vi "timemer.vi"() -> ()   [LabVIEW 2014]
panel:
  out "문자열":string
  in  "확인 버튼 2":bool
  in  "초기화":bool
  in  "확인 버튼":bool
  out "초":i32[](array[numeric])
  out "분":i32[](array[numeric])
  out "시":i32[](array[numeric])
  out "시간":string
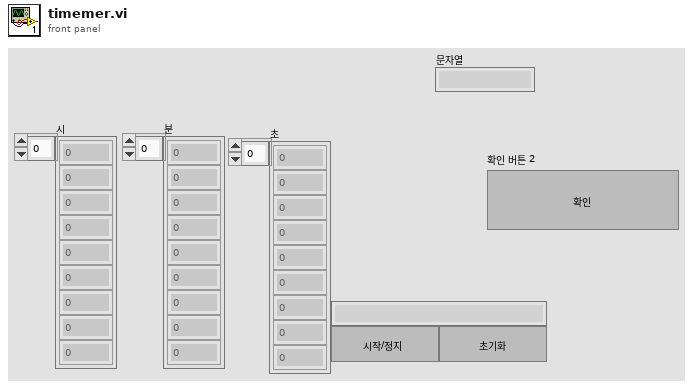
[diagram p1: front panel]
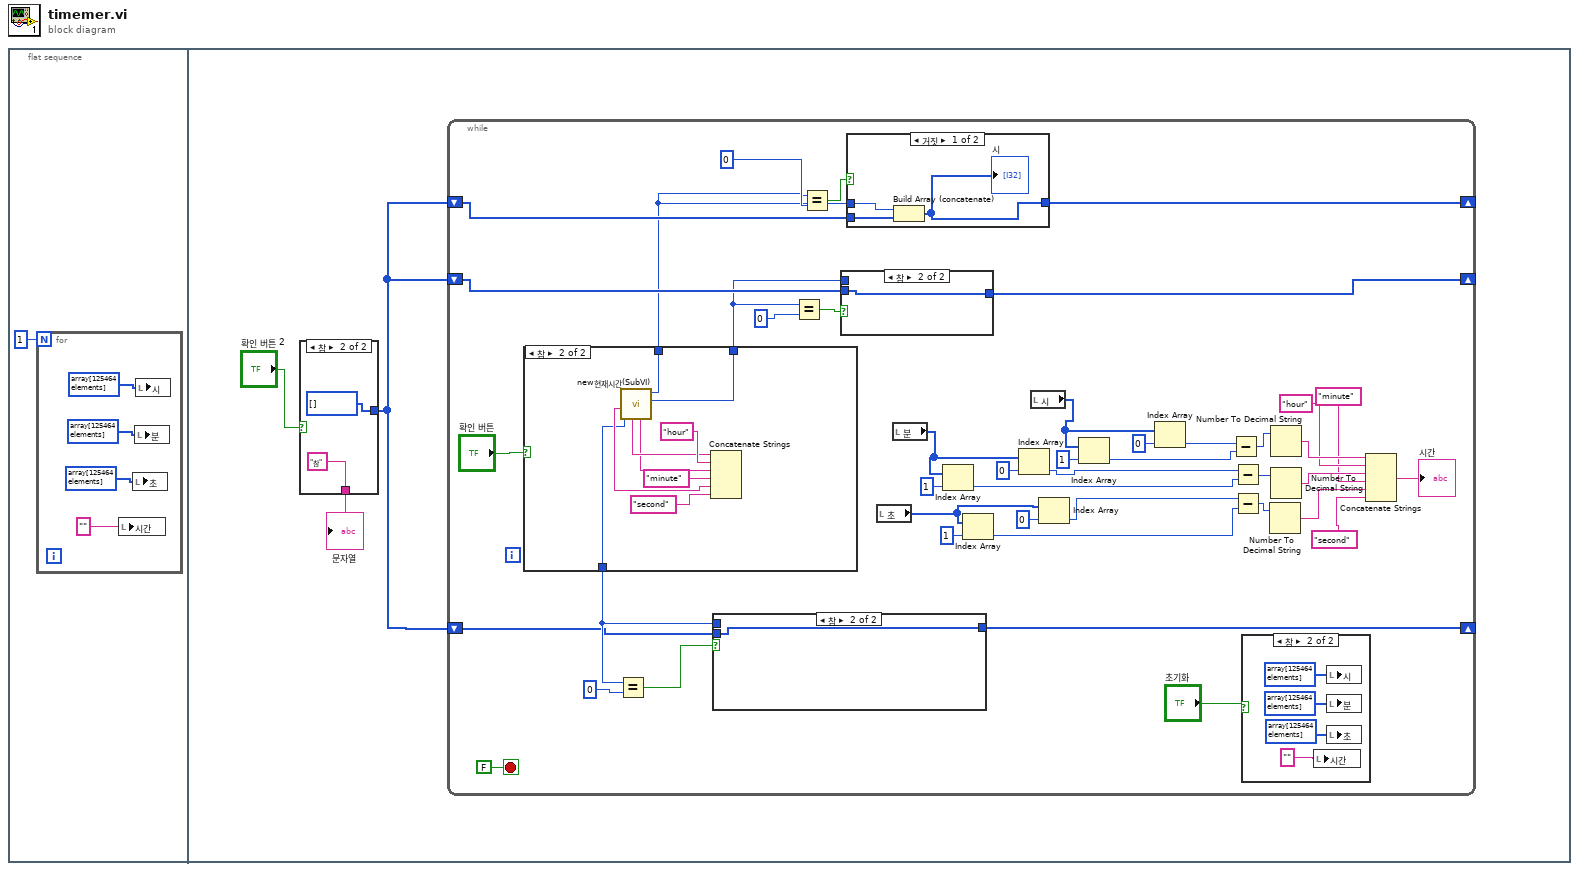
[diagram p0: block diagram]
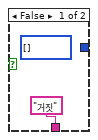
[diagram p2: hidden frame]
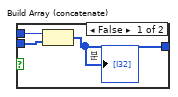
[diagram p5: hidden frame]
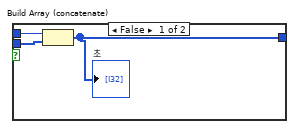
[diagram p6: hidden frame]
diagram:
  n1 = flat-sequence {
    frame #0 {
      n2 = for {
        N: 1 -> [_]
        n3 = local write "시간"("") -> ()
        n4 = local write "초"(i32[] array[125464 elements] ("시")) -> ()
        n5 = local write "분"(i32[] array[125464 elements] ("시")) -> ()
        n6 = local write "시"(i32[] array[125464 elements] ("시")) -> ()
      }
    }
    frame #1 {
      n7 = case shown="참" "확인 버튼 2" {
        tunnel: [_ i32[] []] -> w8
        tunnel: ["거짓" "참"] -> w6
        frame False {
          (unwired) i32[] []
        }
        frame True {
        }
      }
      "문자열" <- w6
      n8 = while "While 루프" {
        shift-right: [w43] -> _
        shift-left: w8 -> [w53]
        shift-right: [w44] -> _
        shift-left: w8 -> [w52]
        shift-right: [w42] -> _
        shift-left: w8 -> [w12]
        stop <- FALSE stop-if-true
        n9 = case shown="참" "확인 버튼" {
          tunnel: [_ w73] -> w50
          tunnel: [_ w72] -> w45
          tunnel: [_ w71] -> w47
          frame False {
          }
          frame True {
            n10 = call "new현재시간(SubVI).vi"() -> ("분"=w71:i32, "시"=w72:i32, "분 문자열"=w75:string, "시 문자열"=w76:string, "초"=w73:i32, "초 문자열"=w74:string)  [unwired: 3 in, 3 out]
            n11 = Concatenate Strings(w76, "hour" ("문자열"), w75, "minute" ("문자열"), w74, "second" ("문자열")) -> ()  [unwired: 1 out]
          }
        }
        n12 = Equal?(x=w50, y=0) -> (x = y?=w41:bool)
        n13 = case shown="참" w41 {
          tunnel: w12 -> [w69 w70]
          tunnel: w50 -> [w68 _]
          tunnel: [w67 w70] -> w42
          frame False {
            n14 = Build Array (concatenate)(w68, w69) -> (w67:i32[])
            "초" <- w67
          }
          frame True {
          }
        }
        n15 = Equal?(x=w47, y=0) -> (x = y?=w40:bool)
        n16 = Equal?(x=w45, y=0) -> (x = y?=w39:bool)
        n17 = case shown="참" w40 {
          tunnel: w52 -> [w65 w66]
          tunnel: w47 -> [w64 _]
          tunnel: [w63 w66] -> w44
          frame False {
            n18 = Build Array (concatenate)(w64, w65) -> (w63:i32[])
            "분" <- w63
          }
          frame True {
          }
        }
        n19 = case shown="거짓" w39 {
          tunnel: w53 -> [w61 w62]
          tunnel: w45 -> [w60 _]
          tunnel: [w59 w62] -> w43
          frame False {
            n20 = Build Array (concatenate)(w60, w61) -> (w59:i32[])
            "시" <- w59
          }
          frame True {
          }
        }
        n21 = local read "초"() -> (w15:i32[])
        n22 = local read "분"() -> (w16:i32[])
        n23 = Index Array(array=w16, index=1 ("인덱스")) -> (element=w22:i32)
        n24 = Index Array(array=w15, index=1 ("인덱스")) -> (element=w18:i32)
        n25 = Index Array(array=w16, index=0 ("인덱스")) -> (element=w23:i32)
        n26 = local read "시"() -> (w17:i32[])
        n27 = Index Array(array=w15, index=0 ("인덱스")) -> (element=w19:i32)
        n28 = Index Array(array=w17, index=1 ("인덱스")) -> (element=w26:i32)
        n29 = Index Array(array=w17, index=0 ("인덱스")) -> (element=w29:i32)
        n30 = Subtract(x=w29, y=w26) -> (x-y=w32:i32)
        n31 = Subtract(x=w23, y=w22) -> (x-y=w31:i32)
        n32 = Subtract(x=w19, y=w18) -> (x-y=w30:i32)
        n33 = case shown="참" "초기화" {
          frame False {
          }
          frame True {
            n34 = local write "시간"("") -> ()
            n35 = local write "시"(i32[] array[125464 elements] ("시")) -> ()
            n36 = local write "분"(i32[] array[125464 elements] ("시")) -> ()
            n37 = local write "초"(i32[] array[125464 elements] ("시")) -> ()
          }
        }
        n38 = Number To Decimal String(number=w30) -> (decimal integer string=w34:string)  [unwired: 1 in]
        n39 = Number To Decimal String(number=w32) -> (decimal integer string=w38:string)  [unwired: 1 in]
        n40 = Number To Decimal String(number=w31) -> (decimal integer string=w36:string)  [unwired: 1 in]
        n41 = Concatenate Strings(w38, "hour" ("문자열"), w36, "minute" ("문자열"), w34, "second" ("문자열")) -> (→"시간":string)
      }
    }
  }
